vi "FindCollectRank.vi"(5 "UID":i32, 9 "VI_AST in":refnum<class "VI_AST.lvclass">) -> (3 "VI_AST out":refnum<class "VI_AST.lvclass">, 4 "collect rank":i32)   [LabVIEW 2014, in "VI_AST.lvclass"]
uses:
  VI_AST.lvclass
  VI_AST.lvclass/VI_AST.ctl
  DAG/DAG/DAG.lvclass/DAG.ctl
  DAG/DAG/DAG.lvclass
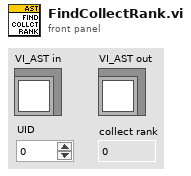
[diagram p1: front panel]
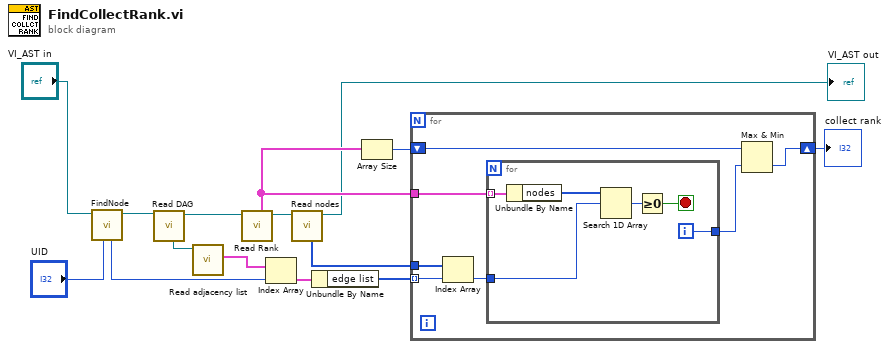
[diagram p0: block diagram]
diagram:
  n1 = call "FindNode.vi"("UID"="UID", "VI_AST in"="VI_AST in") -> ("VI_AST out"=w3:refnum<class "VI_AST.lvclass">, "index"=w7:i32)  [unwired: 6 in]
  n2 = call "Read DAG.vi"("VI_AST in"=w3) -> ("VI_AST out"=w9:refnum<class "VI_AST.lvclass">, "DAG"=w5:refnum<class "DAG.lvclass">)  [unwired: 7 in]
  n3 = call "Read adjacency list.vi"("DAG in"=w5) -> ("adjacency list"=w6:cluster{"edge list":i32[]}[])  [unwired: 9 in, 1 out]
  n4 = call "Read Rank.vi"("VI_AST in"=w9) -> ("VI_AST out"=w10:refnum<class "VI_AST.lvclass">, "Rank"=w14:cluster{"nodes":i32[]}[])  [unwired: 7 in]
  n5 = Index Array(array=w6, index=w7) -> (element=w8:cluster{"edge list":i32[]})
  n6 = call "Read nodes.vi"("VI_AST in"=w10) -> ("VI_AST out"=→"VI_AST out":refnum<class "VI_AST.lvclass">, "nodes"=w11:i32[])  [unwired: 7 in]
  n7 = Unbundle By Name(w8) -> ("edge list"=w12:i32[])
  n8 = Array Size(array=w14) -> (size(s)=w13:i32)
  n9 = for {
    tunnel: w14 -> [w20]
    tunnel: w11 -> [w22]
    tunnel: w12 -> [w21] mode=indexing
    shift-right: [w17] -> w15
    shift-left: w13 -> [w18]
    n10 = Index Array(array=w22, index=w21) -> (element=w19:i32)
    n11 = for {
      tunnel: w20 -> [w28] mode=indexing
      tunnel: w19 -> [w26]
      tunnel: [w23] -> w16
      i -> [w23]
      stop <- w24 stop-if-true
      n12 = Unbundle By Name(w28) -> ("nodes"=w27:i32[])
      n13 = Search 1D Array(1D array=w27, element=w26) -> (index of element=w25:i32)  [unwired: 1 in]
      n14 = Greater Or Equal To 0?(x=w25) -> (x >= 0?=w24:bool)
    }
    n15 = Max & Min(x=w18, y=w16) -> (min(x,y)=w17:i32)  [unwired: 1 out]
  }
  "collect rank" <- w15
